vi "ST_parse_add_part_response.vi"(6 "recordset_in":variant[][](array[variant]), 8 "error_in":errorcluster, 11 "command_nmb":u8) -> (0 "error_out":errorcluster, 3 "reference_data_to_PLC":u8[](array[numeric]))   [LabVIEW 2020]
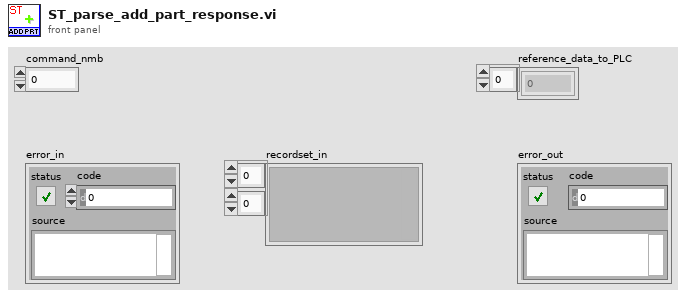
[diagram p1: front panel]
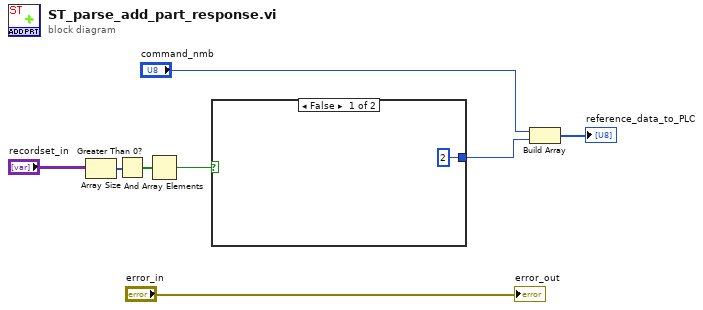
[diagram p0: block diagram]
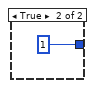
[diagram p2: hidden frame]
diagram:
  n1 = Array Size(array="recordset_in") -> (size(s)=w5:i32[])
  n2 = Greater Than 0?(x=w5) -> (x > 0?=w4:bool[])
  n3 = And Array Elements(Boolean array=w4) -> (logical AND=w1:bool)
  n4 = case shown="False" w1 {
    tunnel: [u8 2 u8 1] -> w6
    frame False {
    }
    frame True {
    }
  }
  n5 = Build Array("command_nmb", w6) -> (→"reference_data_to_PLC":u8[])
  "error_out" <- "error_in"
